vi "Set SubNumber.vi"(8 "error in":errorcluster, 10 "Value":refnum<class "Value.lvclass">, 11 "Object Type in":refnum<class "Object Type Base.lvclass">) -> (0 "error out":errorcluster, 3 "Object Type out":refnum<class "Object Type Base.lvclass">)   [LabVIEW 2019, in "Electronic Datasheet.lvlib" / "Object Type Base.lvclass"]
doc: "Despite for ObjectTypes of Array, SubNumber is not a supported field"
uses:
  Object Type Base.lvclass
  Value/Value.lvclass
  Object Type Base.lvclass/Object Type Base.ctl
  Electronic Datasheet.lvlib
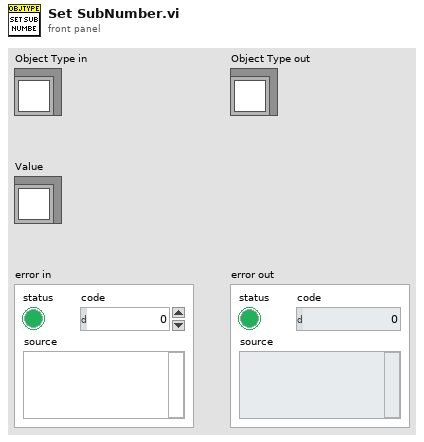
[diagram p1: front panel]
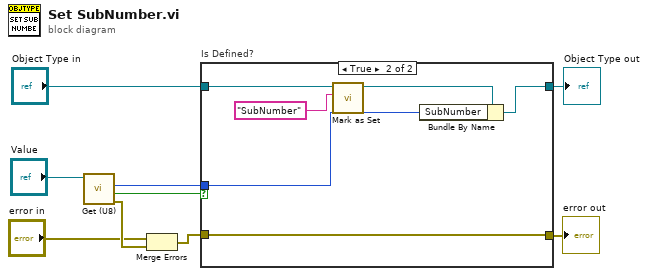
[diagram p0: block diagram]
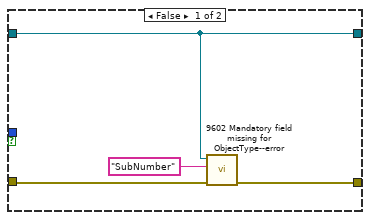
[diagram p2: hidden frame]
diagram:
  n1 = call "Get (U8).vi"("Value in"="Value") -> ("error out"=w4:errorcluster, "Defined?"=w6:bool, "Value"=w3:u8)  [unwired: 7 in, 1 out]
  n2 = Merge Errors("error in", w4) -> (w2:errorcluster)
  n3 = case "Is Defined?" shown="True" w6 {
    tunnel: "Object Type in" -> [w10 w18]
    tunnel: [w10 w17] -> w8
    tunnel: [w12 w19] -> w5
    tunnel: w2 -> [w13 w19]
    tunnel: w3 -> [_ w14]
    frame False {
      n4 = call "9602 Mandatory field missing for ObjectType--error.vi"("error in"=w13, "Field Name"="SubNumber" ("error message (\"\")"), "Object Type Base"=w10) -> ("error out"=w12:errorcluster)  [unwired: 8 in]
    }
    frame True {
      n5 = call "Mark as Set.vi"("Field name"="SubNumber", "Object Type in"=w18) -> ("Object Type out"=w16:refnum<class "Object Type Base.lvclass">)  [unwired: 9 in]
      n6 = Bundle By Name(cluster=w16, "SubNumber"=w14) -> (w17:refnum<class "Object Type Base.lvclass">)
    }
  }
  "Object Type out" <- w8
  "error out" <- w5
